vi "CreateNewWSfile.vi"(4 "reference 5":refnum<vi>, 5 "NewVal":string, 6 "Image":refnum<vi>, 7 "reference in":refnum<vi>, 8 "error in (no error)":errorcluster, 9 "reference 4":refnum<vi>, 10 "reference 3":refnum<vi>, 11 "Path in":refnum<vi>) -> (0 "error out":errorcluster)   [LabVIEW 2013]
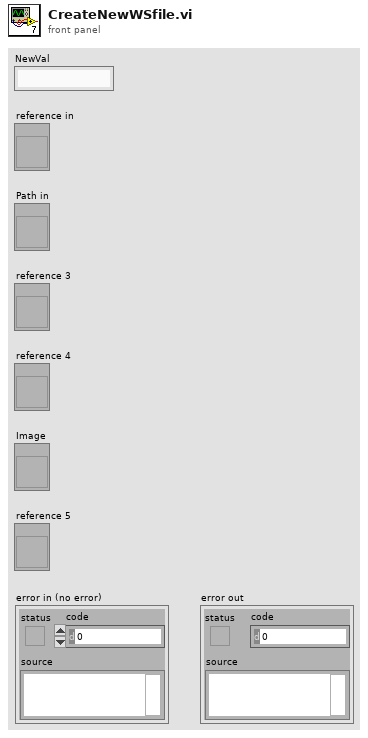
[diagram p1: front panel]
types:
  T1 = enum16{"unknown", "pt3 File", "png Image", "bmp Image"}
  T2 = cluster{"File No":i32, "File Path":path, "Parent File":i32, "File Type":enum16{"unknown", "pt3 File", "png Image", "bmp Image"}, "Measurement Type":enum16{"not a pt3 File", "Image File", "Point Measurement", "Auto Point", "Line Scan", "Grid Scan"}, "Upper Left":cluster{"x-Position":dbl, "y-Position":dbl, "z-Position":dbl}, "Pixels":i32[], "Scan Axis":enum32{"x-y", "x-z", "y-z"}, "Resolution":dbl, "PixelTime":dbl}
  T3 = cluster{"Ident":string, "Format Version":string, "Creator Name":string, "Creator Version":string, "File Time":string, "Comment":string, "Laser":i32, "Binning":i32, "Offset":i32, "AcquisitionTime (ms)":i32, "HardwareSerial":i32, "SyncDivider":i32, "Resolution (ps)":dbl, "Rates":dbl[], "SyncRate":dbl, "CFD Settings":cluster{"Sync Level":i32, "Sync ZeroX":i32, "Sync Offset":i32, "Chan Settings":cluster{"CHx Level":i32, "CHx ZeroX":i32, "CHx Offset":i32}[]}}
  T4 = cluster{"Dimensions":i32, "Time Per Pixel [ms]":dbl, "Acceleration":i32, "Pattern":i32, "X0":sgl, "Y0":sgl, "Z0":dbl, "PixX":i32, "PixY":i32, "PixResol":sgl, "TStartTo":sgl, "TStoptTo":sgl, "TStartFro":sgl, "TStopFro":sgl}
  T5 = enum16{"not a pt3 File", "Image File", "Point Measurement", "Auto Point", "Line Scan", "Grid Scan"}
  T6 = cluster{cluster{"X0":sgl, "Y0":sgl, "Z0":dbl}, "PixX":i32, "PixY":i32, "Pattern":i32, "PixResol":sgl, "Time Per Pixel [ms]":dbl, "Laser":i32}
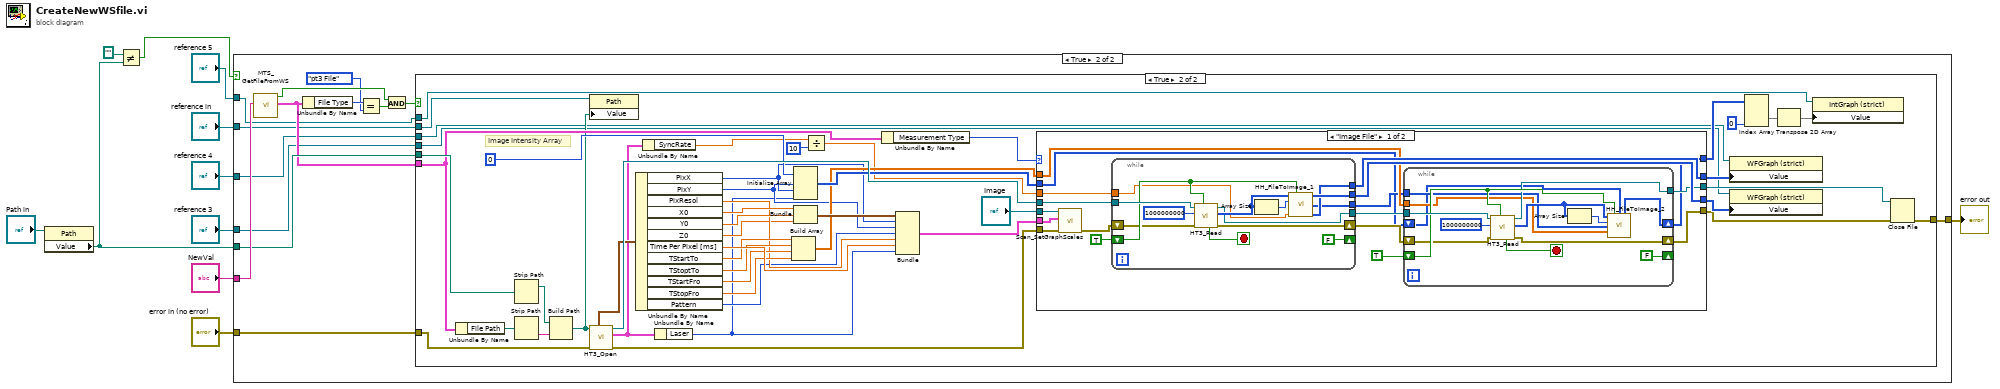
[diagram p0: block diagram]
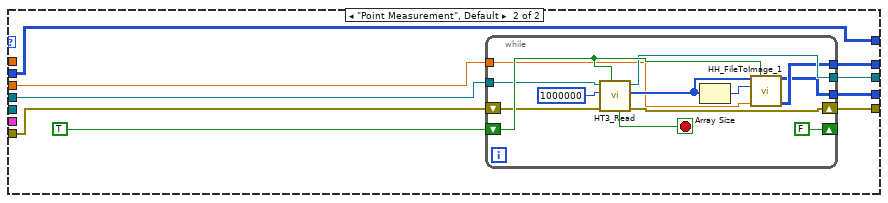
[diagram p4: hidden frame]
diagram:
  n1 = property class="Path"(reference="Path in") -> ("Value"=w10:path)  [unwired: 1 in, 2 out]
  n2 = Not Equal?(x=path "", y=w10) -> (x != y?=w7:bool)
  n3 = case shown="True" w7 {
    tunnel: "NewVal" -> [_ w26]
    tunnel: w10 -> [_ w25]
    tunnel: "error in (no error)" -> [w12 w24]
    tunnel: [w12 w23] -> w9
    tunnel: "reference in" -> [_ w16]
    tunnel: "reference 3" -> [_ w15]
    tunnel: "reference 4" -> [_ w14]
    tunnel: "reference 5" -> [_ w13]
    frame False {
    }
    frame True {
      n4 = call "MTS_GetFileFromWS.vi"("Tree Label"=w26) -> ("File Header"=w22:T2, "File Found"=w21:bool)  [unwired: 9 in]
      n5 = Unbundle By Name(w22) -> ("File Type"=w20:T1)
      n6 = Equal?(x=w20, y=T1."pt3 File" ("File Type")) -> (x = y?=w18:bool)
      n7 = And(x=w21, y=w18) -> (x .and. y?=w17:bool)
      n8 = case shown="True" w17 {
        tunnel: w22 -> [_ w60]
        tunnel: w25 -> [_ w74]
        tunnel: w24 -> [w27 w71]
        tunnel: [w27 w64] -> w23
        tunnel: w16 -> [_ w31]
        tunnel: w15 -> [_ w30]
        tunnel: w14 -> [_ w29]
        tunnel: w13 -> [_ w28]
        frame False {
        }
        frame True {
          # "Image Intensity Array"
          n9 = Unbundle By Name(w60) -> ("File Path"=w73:path)
          n10 = Strip Path(path=w74) -> (stripped path=w72:path)  [unwired: 1 out]
          n11 = Strip Path(path=w73) -> (name=w61:string)  [unwired: 1 out]
          n12 = Build Path(base path=w72, name or relative path=w61) -> (appended path=w54:path)
          n13 = call "HT3_Open.vi"("error in"=w71, "File Path"=w54) -> ("error out"=w70:errorcluster, "Header"=w39:T3, "refnum out"=w69:refnum<file>, "Image Header"=w62:T4)  [unwired: 3 in, 3 out]
          n14 = property class="Path"(reference=w31, "Value"=w54) -> ()  [unwired: 1 in, 2 out]
          n15 = Unbundle By Name(w62) -> ("PixX"=w37:i32, "PixY"=w36:i32, "PixResol"=w43:sgl, "X0"=w56:sgl, "Y0"=w44:sgl, "Z0"=w41:dbl, "Time Per Pixel [ms]"=w53:dbl, "TStartTo"=w50:sgl, "TStoptTo"=w49:sgl, "TStartFro"=w48:sgl, "TStopFro"=w47:sgl, "Pattern"=w40:i32)
          n16 = Unbundle By Name(w39) -> ("SyncRate"=w52:dbl)
          n17 = Unbundle By Name(w39) -> ("Laser"=w32:i32)
          n18 = Build Array(w50, w49, w48, w47) -> (w46:sgl[])
          n19 = Initialize Array(u16 0 ("element"), w36, w37, w32) -> (w57:u16[][][])
          n20 = Bundle("X0"=w56, "Y0"=w44, "Z0"=w41) -> (w55:cluster{"X0":sgl, "Y0":sgl, "Z0":dbl})  [unwired: 1 in]
          n21 = Divide(x=w52, y=10) -> (x/y=w45:dbl)
          n22 = Unbundle By Name(w60) -> ("Measurement Type"=w59:T5)
          n23 = Bundle(w55, "PixX"=w37, "PixY"=w36, "Pattern"=w40, "PixResol"=w43, "Time Per Pixel [ms]"=w53, "Laser"=w32) -> (w63:T6)  [unwired: 1 in]
          n24 = case shown="\"Image File\"" w59 {
            tunnel: w70 -> [w88 w128]
            tunnel: w69 -> [w91 w127]
            tunnel: [w90 w123] -> w68
            tunnel: [w89 w124] -> w67
            tunnel: [w80 w126] -> w66
            tunnel: [w82 w125] -> w65
            tunnel: "Image" -> [w87 _]
            tunnel: w63 -> [w86 _]
            tunnel: w57 -> [w76 w122]
            tunnel: w45 -> [w79 w121]
            tunnel: w46 -> [w78 _]
            tunnel: [w75 w122] -> w38
            frame "Image File" {
              n25 = call "Scan_SetGraphScales.vi"("error in (no error)"=w88, "Image Measurent Parameters"=w86, "Image"=w87) -> ("error out"=w85:errorcluster)  [unwired: 8 in]
              n26 = while {
                tunnel: w91 -> [w120]
                shift-right: [FALSE ("Start From Top")] -> _
                shift-left: TRUE ("Start From Top") -> [w115]
                shift-right: [w114] -> w83
                shift-left: w85 -> [w111]
                tunnel: [w113] -> w81
                tunnel: [w112] -> w90
                tunnel: [w110] -> w89
                tunnel: w79 -> [w109]
                tunnel: [w107] -> w77
                stop <- w117 stop-if-true
                n27 = call "HT3_Read.vi"("Start From Top"=w115, "error in"=w111, "Data count"=1000000000, "refnum in"=w120) -> ("error out"=w114:errorcluster, "Data out"=w116:u32[], "refnum out"=w113:refnum<file>, "EOF?"=w117:bool)  [unwired: 4 in]
                n28 = Array Size(array=w116) -> (size(s)=w108:i32)
                n29 = call "HH_FileToImage_1.vi"("Data In"=w116, "Reset"=w115, "Data Count"=w108, "Trace Bins"=w109) -> ("Histograms"=w112:i32[][], "Trigger Times"=w107:u64[], "Traces"=w110:i32[][])  [unwired: 6 in, 3 out]
              }
              n30 = while {
                tunnel: w81 -> [w106]
                shift-right: [FALSE ("Start From Top")] -> _
                shift-left: TRUE ("Start From Top") -> [w101]
                shift-right: [w100] -> w82
                shift-left: w83 -> [w98]
                tunnel: [w99] -> w80
                tunnel: w78 -> [w96]
                tunnel: w77 -> [w95]
                shift-right: [w93] -> w75
                shift-left: w76 -> [w94]
                stop <- w103 stop-if-true
                n31 = call "HT3_Read.vi"("Start From Top"=w101, "error in"=w98, "Data count"=1000000000, "refnum in"=w106) -> ("error out"=w100:errorcluster, "Data out"=w102:u32[], "refnum out"=w99:refnum<file>, "EOF?"=w103:bool)  [unwired: 4 in]
                n32 = Array Size(array=w102) -> (size(s)=w97:i32)
                n33 = call "HH_FileToImage_2.vi"("Data In"=w102, "Reset"=w101, "Image Data In"=w94, "Data Count"=w97, "Trigger Times"=w95, "Trigger"=w96) -> ("Image Data Out"=w93:u16[][][])  [unwired: 6 in, 3 out]
              }
            }
            frame "Point Measurement", Default {
              n34 = while {
                tunnel: w127 -> [w140]
                tunnel: [w139] -> w126
                tunnel: [w135] -> w124
                tunnel: [w134] -> w123
                shift-right: [FALSE] -> _
                shift-left: TRUE ("Start From Top") -> [w142]
                tunnel: w121 -> [w131]
                shift-right: [w138] -> w125
                shift-left: w128 -> [w141]
                stop <- w132 stop-if-true
                n35 = call "HT3_Read.vi"("Start From Top"=w142, "error in"=w141, "Data count"=1000000, "refnum in"=w140) -> ("error out"=w138:errorcluster, "Data out"=w136:u32[], "refnum out"=w139:refnum<file>, "EOF?"=w132:bool)  [unwired: 4 in]
                n36 = Array Size(array=w136) -> (size(s)=w130:i32)
                n37 = call "HH_FileToImage_1.vi"("Data In"=w136, "Reset"=w142, "Data Count"=w130, "Trace Bins"=w131) -> ("Histograms"=w134:i32[][], "Traces"=w135:i32[][])  [unwired: 6 in, 4 out]
              }
            }
          }
          n38 = property class="WFGraph (strict)"(reference=w29, "Value"=w67) -> ()  [unwired: 1 in, 2 out]
          n39 = property class="WFGraph (strict)"(reference=w30, "Value"=w68) -> ()  [unwired: 1 in, 2 out]
          n40 = Index Array(array=w38, index (dim 2)=0) -> (element=w35:u16[][])  [unwired: 2 in]
          n41 = Transpose 2D Array(2D array=w35) -> (transposed array=w33:u16[][])
          n42 = property class="IntGraph (strict)"(reference=w28, "Value"=w33) -> ()  [unwired: 1 in, 2 out]
          n43 = Close File(refnum=w66, error in=w65) -> (error out=w64:errorcluster)  [unwired: 1 out]
        }
      }
    }
  }
  "error out" <- w9
